vi "Strain Configure Full Bridge Poisson.vi"(0 "instrument handle":refnum<k15>, 1 "Range":dbl, 2 "SampTime":dbl, 5 "GaugeFactor":dbl, 7 "PoissonRatio":dbl, 9 "ExcitationVoltage":dbl, 11 "error in (no error)":errorcluster {"code" format="%.0x"}, 12 "SampCount":i32 format="%.0g", 13 "Channel":string) -> (4 "instrument handle out":refnum<k15>, 15 "error out":errorcluster {"code" format="%.0x"})   [LabVIEW 2020, in "Keysight DAQ970.lvlib"]
doc: "Configures a specified channel for full Poisson bridge strain gauge DMM digitizing, but they do not initiate the digitizing. This command redefines the scan list."
uses:
  Keysight DAQ970.lvlib
  KtDAQ970.dll
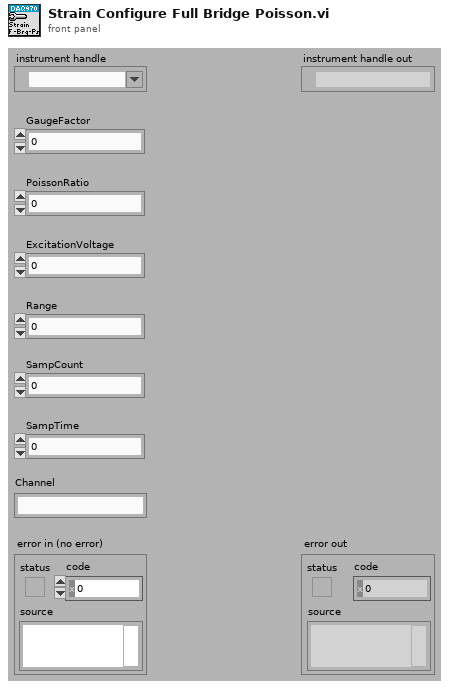
[diagram p1: front panel]
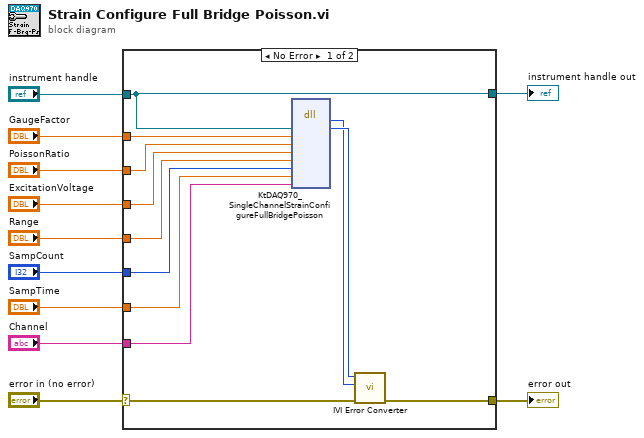
[diagram p0: block diagram]
diagram:
  n1 = case shown="No Error" "error in (no error)" {
    selector: "error in (no error)" -> [w21 w25]
    tunnel: [w20 w25] -> w11
    tunnel: "instrument handle" -> [w12 w24]
    tunnel: "GaugeFactor" -> [w19 _]
    tunnel: "PoissonRatio" -> [w18 _]
    tunnel: "ExcitationVoltage" -> [w17 _]
    tunnel: "Range" -> [w16 _]
    tunnel: "SampCount" -> [w15 _]
    tunnel: "SampTime" -> [w14 _]
    tunnel: "Channel" -> [w13 _]
    tunnel: [w12 w24] -> w1
    frame No Error {
      n2 = dll-call lib="KtDAQ970**.dll" fn="KtDAQ970_SingleChannelStrainConfigureFullBridgePoisson"("Vi"=w12, "GaugeFactor"=w19, "PoissonRatio"=w18, "ExcitationVoltage"=w17, "Range"=w16, "SampCount"=w15, "SampTime"=w14, "Channel"=w13) -> (w22:i32, "Vi"=w23:u32)  [unwired: 10 in, 2 out]
      n3 = call "IVI Error Converter.vi"("error in (no error)"=w21, "IVI error code (0)"=w22, "instrument handle"=w23) -> ("error out"=w20:errorcluster)  [unwired: 7 in, 1 out]
    }
    frame Error {
    }
  }
  "error out" <- w11
  "instrument handle out" <- w1
